vi "Check D_Tunnel on Server.vi"(0 "Values":dbl[](array[numeric]) format="%.2f", 2 "Ch Names":string[](array[string]), 3 "Current Time":dbl format="%.2f", 4 "Adam Loop Count":i32) -> (6 "Scan comment":string)   [LabVIEW 2022 SP3]
uses:
  Anemometry/Anemometry Sub Vis/Controls/In_Range.ctl
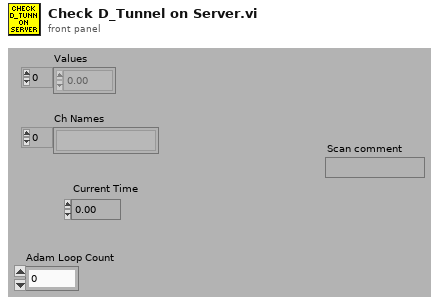
[diagram p1: front panel]
types:
  T1 = typedef "In_Range.ctl" = enum16{"%", "±", "% & ±"}
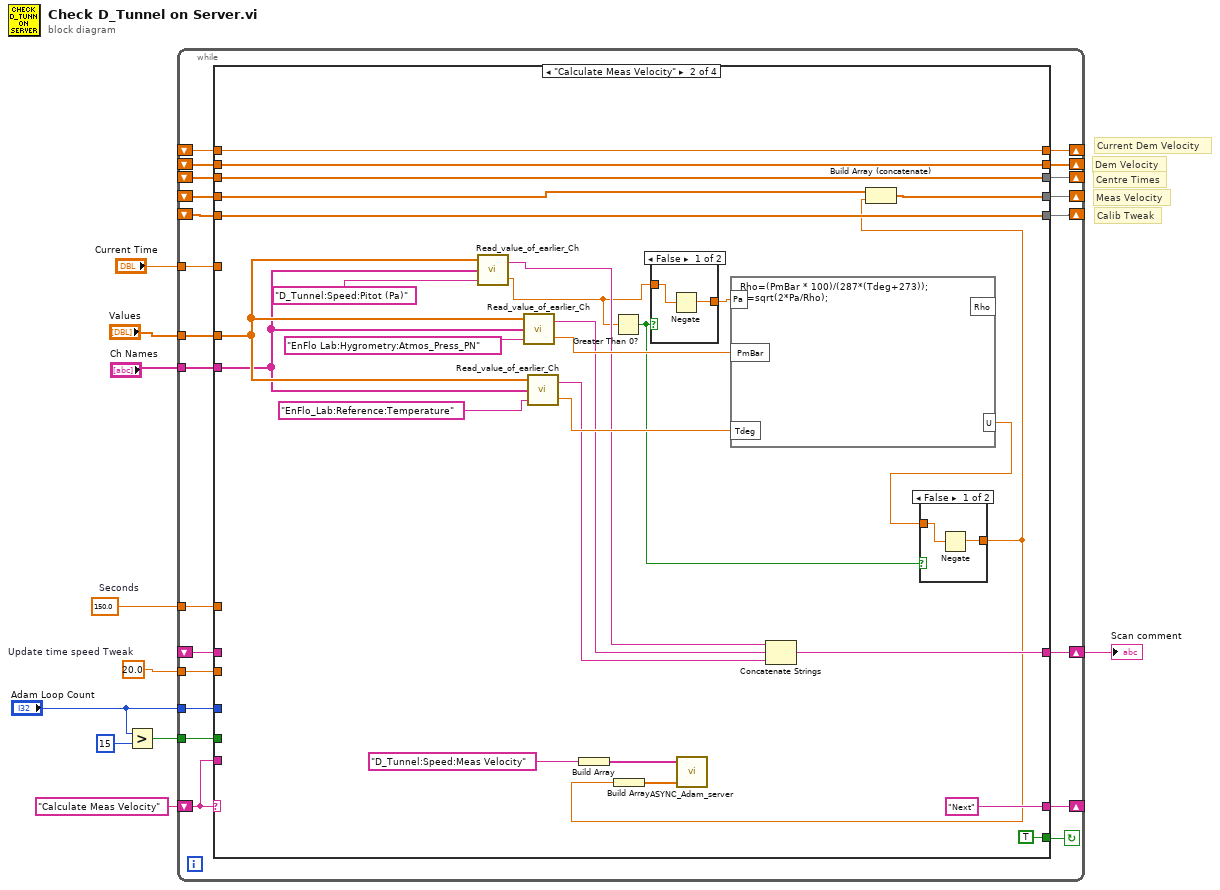
[diagram p0: block diagram]
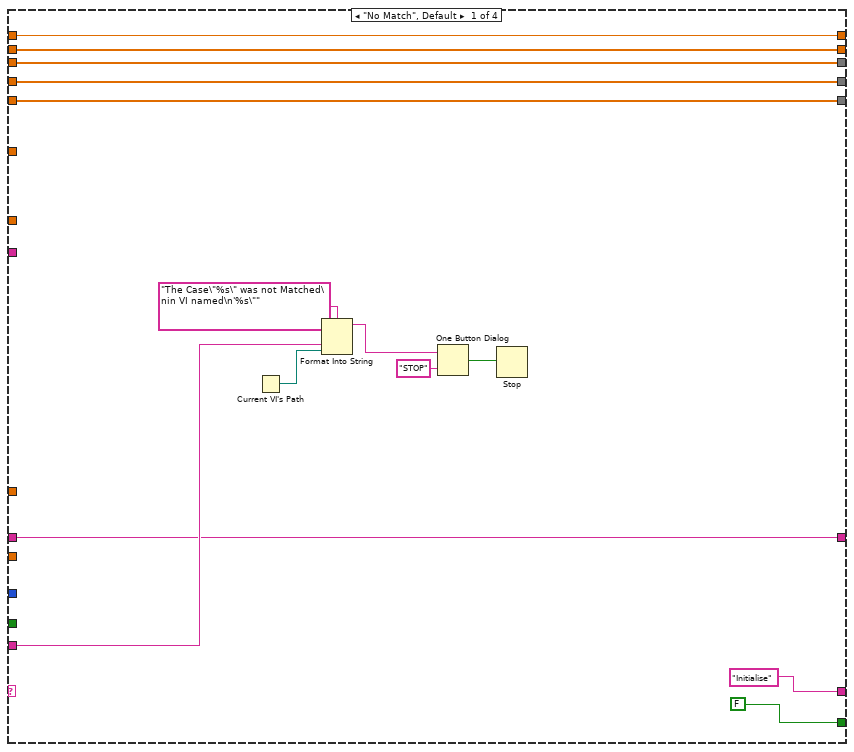
[diagram p2: hidden frame]
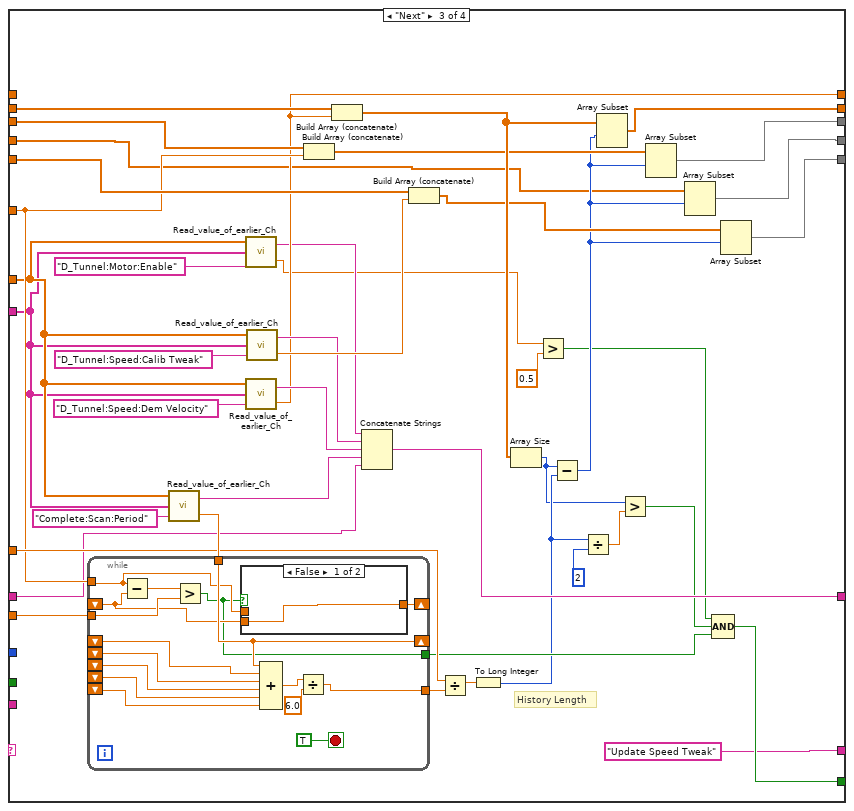
[diagram p5: hidden frame]
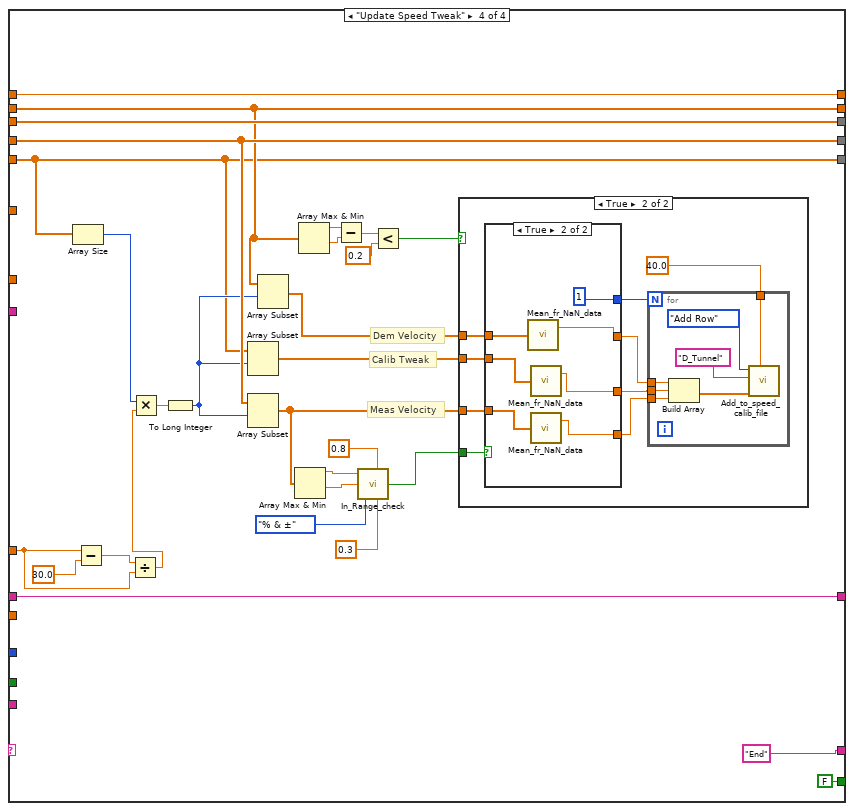
[diagram p7: hidden frame]
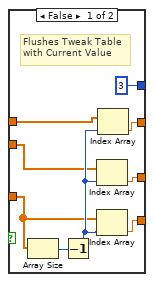
[diagram p9: hidden frame]
diagram:
  w3 = 20.0  # Update time speed Tweak
  w4 = 150.0  # Seconds
  # "Calib Tweak"
  # "Meas Velocity"
  # "Dem Velocity"
  # "Centre Times"
  # "Current Dem Velocity"
  n1 = Greater?(x="Adam Loop Count", y=15) -> (0:w6:bool)
  n2 = while {
    shift-left: "Calculate Meas Velocity" ("t") -> [w30]
    shift-right: [w31] -> _
    tunnel: "Values" -> [w29]
    tunnel: "Ch Names" -> [w28]
    shift-right: [w27] -> _
    shift-left: _ -> [w26]
    shift-right: [w24] -> _
    shift-left: _ -> [w25]
    shift-right: [w21] -> _
    shift-left: _ -> [w22]
    tunnel: "Current Time" -> [w23]
    tunnel: w6 -> [w20]
    shift-right: [w19] -> w5
    shift-left: _ -> [w18]
    tunnel: w4 -> [w17]
    shift-right: [w16] -> _
    shift-left: _ -> [w15]
    shift-right: [w14] -> _
    shift-left: _ -> [w13]
    tunnel: w3 -> [w12]
    tunnel: "Adam Loop Count" -> [w11]
    stop <- w32 continue-if-true
    n3 = case shown="\"Calculate Meas Velocity\"" w30 {
      tunnel: [FALSE TRUE w81 FALSE] -> w32
      tunnel: ["Initialise" "Next" ("t") "Update Speed Tweak" ("t") "End" ("t")] -> w31
      tunnel: w30 -> [w41 _ _ _]
      tunnel: w29 -> [_ w53 w90 _]
      tunnel: w28 -> [_ w52 w89 _]
      tunnel: [w38 w69 w97 w168] -> w27
      tunnel: w26 -> [w38 w69 _ w168]
      tunnel: w25 -> [w37 w68 w119 w144]
      tunnel: [w37 w68 w117 w144] -> w24
      tunnel: w23 -> [_ _ w102 _]
      tunnel: w22 -> [w36 w67 w115 w167]
      tunnel: [w36 w67 w114 w167] -> w21
      tunnel: w20 -> [_ _ _ _]
      tunnel: [w35 w57 w112 w166] -> w19
      tunnel: w18 -> [w35 _ w83 w166]
      tunnel: w17 -> [_ _ w111 w163]
      tunnel: [w34 w70 w104 w156] -> w16
      tunnel: w15 -> [w34 w72 w84 w156]
      tunnel: [w33 w66 w103 w142] -> w14
      tunnel: w13 -> [w33 w66 w106 w142]
      tunnel: w12 -> [_ _ w101 _]
      tunnel: w11 -> [_ _ _ _]
      frame "No Match", Default {
        n4 = Current VI's Path() -> (path=w40:path)
        n5 = Format Into String(format string="The Case\"%s\" was not Matched\nin VI named\n'%s\"" ("Format String"), w41, w40) -> (resulting string=w44:string)  [unwired: 2 in, 1 out]
        n6 = One Button Dialog(message=w44, button name ("OK")="STOP") -> (true=w42:bool)
        n7 = Stop(stop? (T)=w42) -> ()
      }
      frame "Calculate Meas Velocity" {
        n8 = call "Read_value_of_earlier_Ch.vi"("Desired Ch to Read"="D_Tunnel:Speed:Pitot (Pa)", "Ch names"=w52, "Present scan array"=w53) -> ("Value"=w51:dbl, "Scan comment"=w60:string)  [unwired: 1 in]
        n9 = call "Read_value_of_earlier_Ch.vi"("Desired Ch to Read"="EnFlo Lab:Hygrometry:Atmos_Press_PN", "Ch names"=w52, "Present scan array"=w53) -> ("Value"=w62:dbl, "Scan comment"=w59:string)  [unwired: 1 in]
        n10 = call "Read_value_of_earlier_Ch.vi"("Desired Ch to Read"="EnFlo_Lab:Reference:Temperature", "Ch names"=w52, "Present scan array"=w53) -> ("Value"=w61:dbl, "Scan comment"=w58:string)  [unwired: 1 in]
        n11 = Build Array("D_Tunnel:Speed:Meas Velocity") -> (w56:string[])
        n12 = Greater Than 0?(x=w51) -> (x > 0?=w48:bool)
        n13 = case shown="False" w48 {
          tunnel: [w77 w79] -> w50
          tunnel: w51 -> [w78 w79]
          frame False {
            n14 = Negate(x=w78) -> (-x=w77:dbl)
          }
          frame True {
          }
        }
        n15 = formula code="Rho=(PmBar * 100)/(287*(Tdeg+273));\nU=sqrt(2*Pa/Rho);"("Pa"=w50, "Tdeg"=w61, "PmBar"=w62) -> ("U"=w49:dbl)  [unwired: 1 out]
        n16 = Concatenate Strings(w60, w59, w58) -> (w57:string)
        n17 = case shown="False" w48 {
          tunnel: [w74 w76] -> w47
          tunnel: w49 -> [w75 w76]
          frame False {
            n18 = Negate(x=w75) -> (-x=w74:dbl)
          }
          frame True {
          }
        }
        n19 = Build Array(w47) -> (w55:dbl[])
        n20 = call "ASYNC_Adam_server.vi"("Values"=w55, "Channel Names"=w56) -> ()  [unwired: 1 in, 3 out]
        n21 = Build Array (concatenate)(w72, w47) -> (w70:dbl[])
      }
      frame "Next" {
        # "History Length"
        n22 = call "Read_value_of_earlier_Ch.vi"("Desired Ch to Read"="Complete:Scan:Period", "Ch names"=w89, "Present scan array"=w90) -> ("Value"=w121:dbl, "Scan comment"=w113:string)  [unwired: 1 in]
        n23 = while {
          shift-right: [w138] -> _
          shift-left: _ -> [w137]
          tunnel: w121 -> [w138]
          shift-left: _ -> [w136]
          shift-left: _ -> [w135]
          shift-left: _ -> [w134]
          shift-left: _ -> [w133]
          tunnel: [w129] -> w120
          tunnel: w102 -> [w125]
          shift-right: [w126] -> _
          shift-left: _ -> [w124]
          tunnel: w101 -> [w127]
          tunnel: [w123] -> w100
          stop <- TRUE stop-if-true
          n24 = Subtract(x=w125, y=w124) -> (x-y=w128:dbl)
          n25 = Greater?(x=w128, y=w127) -> (0:w123:bool)
          n26 = case shown="False" w123 {
            tunnel: [w139 w140] -> w126
            tunnel: w125 -> [_ w140]
            tunnel: w124 -> [w139 _]
            frame False {
            }
            frame True {
            }
          }
          n27 = Compound Arithmetic op=ADD(w138, w137, w136, w135, w134, w133) -> (w131:dbl)
          n28 = Divide(x=w131, y=6.0) -> (x/y=w129:dbl)
        }
        n29 = call "Read_value_of_earlier_Ch.vi"("Desired Ch to Read"="D_Tunnel:Motor:Enable", "Ch names"=w89, "Present scan array"=w90) -> ("Value"=w86:dbl, "Scan comment"=w87:string)  [unwired: 1 in]
        n30 = call "Read_value_of_earlier_Ch.vi"("Desired Ch to Read"="D_Tunnel:Speed:Dem Velocity", "Ch names"=w89, "Present scan array"=w90) -> ("Value"=w97:dbl, "Scan comment"=w98:string)  [unwired: 1 in]
        n31 = call "Read_value_of_earlier_Ch.vi"("Desired Ch to Read"="D_Tunnel:Speed:Calib Tweak", "Ch names"=w89, "Present scan array"=w90) -> ("Value"=w107:dbl, "Scan comment"=w99:string)  [unwired: 1 in]
        n32 = Build Array (concatenate)(w115, w102) -> (w108:dbl[])
        n33 = Build Array (concatenate)(w119, w97) -> (w116:dbl[])
        n34 = Concatenate Strings(w87, w99, w98, w113, w83) -> (w112:string)
        n35 = Build Array (concatenate)(w106, w107) -> (w105:dbl[])
        n36 = Divide(x=w111, y=w120) -> (x/y=w118:dbl)
        n37 = To Long Integer(number=w118) -> (32bit integer=w95:i32)
        n38 = Array Size(array=w116) -> (size(s)=w94:i32)
        n39 = Greater?(x=w86, y=0.5) -> (0:w82:bool)
        n40 = Subtract(x=w94, y=w95) -> (x-y=w91:i32)
        n41 = Divide(x=w95, y=2) -> (x/y=w93:dbl)
        n42 = Array Subset(array=w116, index=w91) -> (w117:dbl[])  [unwired: 1 in]
        n43 = Greater?(x=w94, y=w93) -> (0:w92:bool)
        n44 = Array Subset(array=w108, index=w91) -> (w114:dbl[])  [unwired: 1 in]
        n45 = Array Subset(array=w84, index=w91) -> (w104:dbl[])  [unwired: 1 in]
        n46 = Compound Arithmetic op=AND(w82, w92, w100) -> (w81:bool)
        n47 = Array Subset(array=w105, index=w91) -> (w103:dbl[])  [unwired: 1 in]
      }
      frame "Update Speed Tweak" {
        # "Meas Velocity"
        # "Calib Tweak"
        # "Dem Velocity"
        n48 = Array Size(array=w142) -> (size(s)=w141:i32)
        n49 = Subtract(x=w163, y=30.0) -> (x-y=w164:dbl)
        n50 = Divide(x=w164, y=w163) -> (x/y=w162:dbl)
        n51 = Multiply(x=w141, y=w162) -> (x*y=w161:dbl)
        n52 = To Long Integer(number=w161) -> (32bit integer=w154:i32)
        n53 = Array Subset(array=w142, index=w154) -> (w152:dbl[])  [unwired: 1 in]
        n54 = Array Subset(array=w156, index=w154) -> (w151:dbl[])  [unwired: 1 in]
        n55 = Array Subset(array=w144, index=w154) -> (w153:dbl[])  [unwired: 1 in]
        n56 = Array Max & Min(array=w151) -> (max value=w150:dbl, min value=w149:dbl)  [unwired: 2 out]
        n57 = Array Max & Min(array=w144) -> (max value=w160:dbl, min value=w159:dbl)  [unwired: 2 out]
        n58 = Subtract(x=w160, y=w159) -> (x-y=w158:dbl)
        n59 = call "In_Range_check.vi"("±"=0.3, "%"=0.8, "Mode"=In_Range."% & ±", "Value"=w149, "Setpoint"=w150) -> ("In Range"=w145:bool)  [unwired: 2 out]
        n60 = Less?(x=w158, y=0.2) -> (x < y?=w155:bool)
        n61 = case shown="True" w155 {
          tunnel: w153 -> [_ w178]
          tunnel: w152 -> [_ w177]
          tunnel: w151 -> [_ w176]
          tunnel: w145 -> [_ w172]
          frame False {
          }
          frame True {
            n62 = case shown="True" w172 {
              tunnel: w178 -> [w192 w201]
              tunnel: w177 -> [w191 w200]
              tunnel: w176 -> [w190 w199]
              tunnel: [w189 w198] -> w175
              tunnel: [w188 w197] -> w174
              tunnel: [w187 w196] -> w173
              tunnel: [3 1] -> w171
              frame False {
                # "Flushes Tweak Table\nwith Current Value"
                n63 = Array Size(array=w190) -> (size(s)=w194:i32)
                n64 = Decrement(x=w194) -> (x-1=w193:i32)
                n65 = Index Array(array=w191, index=w193) -> (element=w188:dbl)
                n66 = Index Array(array=w190, index=w193) -> (element=w189:dbl)
                n67 = Index Array(array=w192, index=w193) -> (element=w187:dbl)
              }
              frame True {
                n68 = call "Mean_fr_NaN_data.vi"("Data"=w201) -> ("Mean value"=w196:dbl)  [unwired: 1 out]
                n69 = call "Mean_fr_NaN_data.vi"("Data"=w200) -> ("Mean value"=w197:dbl)  [unwired: 1 out]
                n70 = call "Mean_fr_NaN_data.vi"("Data"=w199) -> ("Mean value"=w198:dbl)  [unwired: 1 out]
              }
            }
            n71 = for {
              N: w171 -> [_]
              tunnel: w175 -> [w182]
              tunnel: w174 -> [w181]
              tunnel: w173 -> [w180]
              tunnel: 40.0 ("Max Velocity") -> [w179]
              n72 = Build Array(w180, w181, w182) -> (w183:dbl[])
              n73 = call "Add_to_speed_calib_file.vi"("Max Velocity"=w179, "New Row"=w183, "Rig Name"="D_Tunnel" ("y"), "Mode"=enum16{"Add Row", "Get Error Value"}."Add Row") -> ()  [unwired: 2 in, 2 out]
            }
          }
        }
      }
    }
  }
  "Scan comment" <- w5
